vi "Experiment header-Save_Load config file data.vi"(5 "Header file actions":T1=enum."Write All", 7 "Header file sections":T19=enum."LOGIN", 8 "error in (no error)":errorcluster, 9 "All header parameters in":T2 {"VOLUME IMAGING"."Plane Mode" items=["XY Plane", "XZ Plane", "YZ Plane", "arbitraryplane"]; "VOLUME IMAGING"."Basic Image meta data"."Frame Size" items=["100X100"=100, "128X128"=128, "200X200"=200, "256X256"=256, "512X512"=512, "1024x1024"=1024, "2048x2048"=2048]; "AOL Z-STACK"."Hdr Basic Image meta data"."Frame Size" items=["100X100"=100, "128X128"=128, "200X200"=200, "256X256"=256, "512X512"=512, "1024x1024"=1024, "2048x2048"=2048]; "MOTOR Z-STACK"."Hdr Basic Image meta data"."Frame Size" items=["100X100"=100, "128X128"=128, "200X200"=200, "256X256"=256, "512X512"=512, "1024x1024"=1024, "2048x2048"=2048]; "FUNCTIONAL IMAGING"."Plane Mode" items=["XY Plane", "XZ Plane", "YZ Plane", "arbitraryplane"]; "FUNCTIONAL IMAGING"."Basic Image meta data"."Frame Size" items=["100X100"=100, "128X128"=128, "200X200"=200, "256X256"=256, "512X512"=512, "1024x1024"=1024, "2048x2048"=2048]; "TIME SERIES"."Basic Image meta data"."Frame Size" items=["100X100"=100, "128X128"=128, "200X200"=200, "256X256"=256, "512X512"=512, "1024x1024"=1024, "2048x2048"=2048]}, 11 "Experiment data folder path":path) -> (0 "error out":errorcluster, 1 "All header parameters out":T2 {"VOLUME IMAGING"."Plane Mode" items=["XY Plane", "XZ Plane", "YZ Plane", "arbitraryplane"]; "VOLUME IMAGING"."Basic Image meta data"."Frame Size" items=["100X100"=100, "128X128"=128, "200X200"=200, "256X256"=256, "512X512"=512, "1024x1024"=1024, "2048x2048"=2048]; "AOL Z-STACK"."Hdr Basic Image meta data"."Frame Size" items=["100X100"=100, "128X128"=128, "200X200"=200, "256X256"=256, "512X512"=512, "1024x1024"=1024, "2048x2048"=2048]; "MOTOR Z-STACK"."Hdr Basic Image meta data"."Frame Size" items=["100X100"=100, "128X128"=128, "200X200"=200, "256X256"=256, "512X512"=512, "1024x1024"=1024, "2048x2048"=2048]; "FUNCTIONAL IMAGING"."Plane Mode" items=["XY Plane", "XZ Plane", "YZ Plane", "arbitraryplane"]; "FUNCTIONAL IMAGING"."Basic Image meta data"."Frame Size" items=["100X100"=100, "128X128"=128, "200X200"=200, "256X256"=256, "512X512"=512, "1024x1024"=1024, "2048x2048"=2048]; "TIME SERIES"."Basic Image meta data"."Frame Size" items=["100X100"=100, "128X128"=128, "200X200"=200, "256X256"=256, "512X512"=512, "1024x1024"=1024, "2048x2048"=2048]})   [LabVIEW 2017]
doc: "This self-contained module handles all header files save/write operations.\nIt can generate a number of different header files containing different parameters.\nEach different type of header file has its own type defined cluster of parameters.\nThe functionality is fully self-scalable such as when new parameters are added or parameters are deleted or renamed in the typedef clusters this is all handled automatically without the need for further updates to this module."
uses:
  Typedefs/Header parameters cluster-ALL.ctl
  Typedefs/Header subclusters/Header params -Login.ctl
  Typedefs/Header subclusters/Header params-Global Parameters.ctl
  Misc/Experiment Type.ctl
  Typedefs/Header subclusters/Header params-Imaging Modes.ctl
  Typedefs/Header subclusters/Header params-Time Series.ctl
  Typedefs/Header subclusters/Header params-Basic image meta data.ctl
  Typedefs/Frame Size.ctl
  Typedefs/Header subclusters/Header params-Motor Z-stack.ctl
  Typedefs/Header subclusters/Header params-AOL Z-stack.ctl
  Typedefs/Header subclusters/Header params-Functional Imaging.ctl
  Typedefs/Functional Mode.ctl
  Typedefs/AOL modes.ctl
  Typedefs/Plane Mode.ctl
  Typedefs/Header subclusters/Header params-Calibration Setup.ctl
  Typedefs/Header subclusters/Header params-statistics.ctl
  Misc/Biology Information.ctl
  Typedefs/Header file sections.ctl
  Typedefs/Header file actions.ctl
panel:
  out "error":errorcluster
  # "Actual FOV ------>\n(not norm FOFV)"
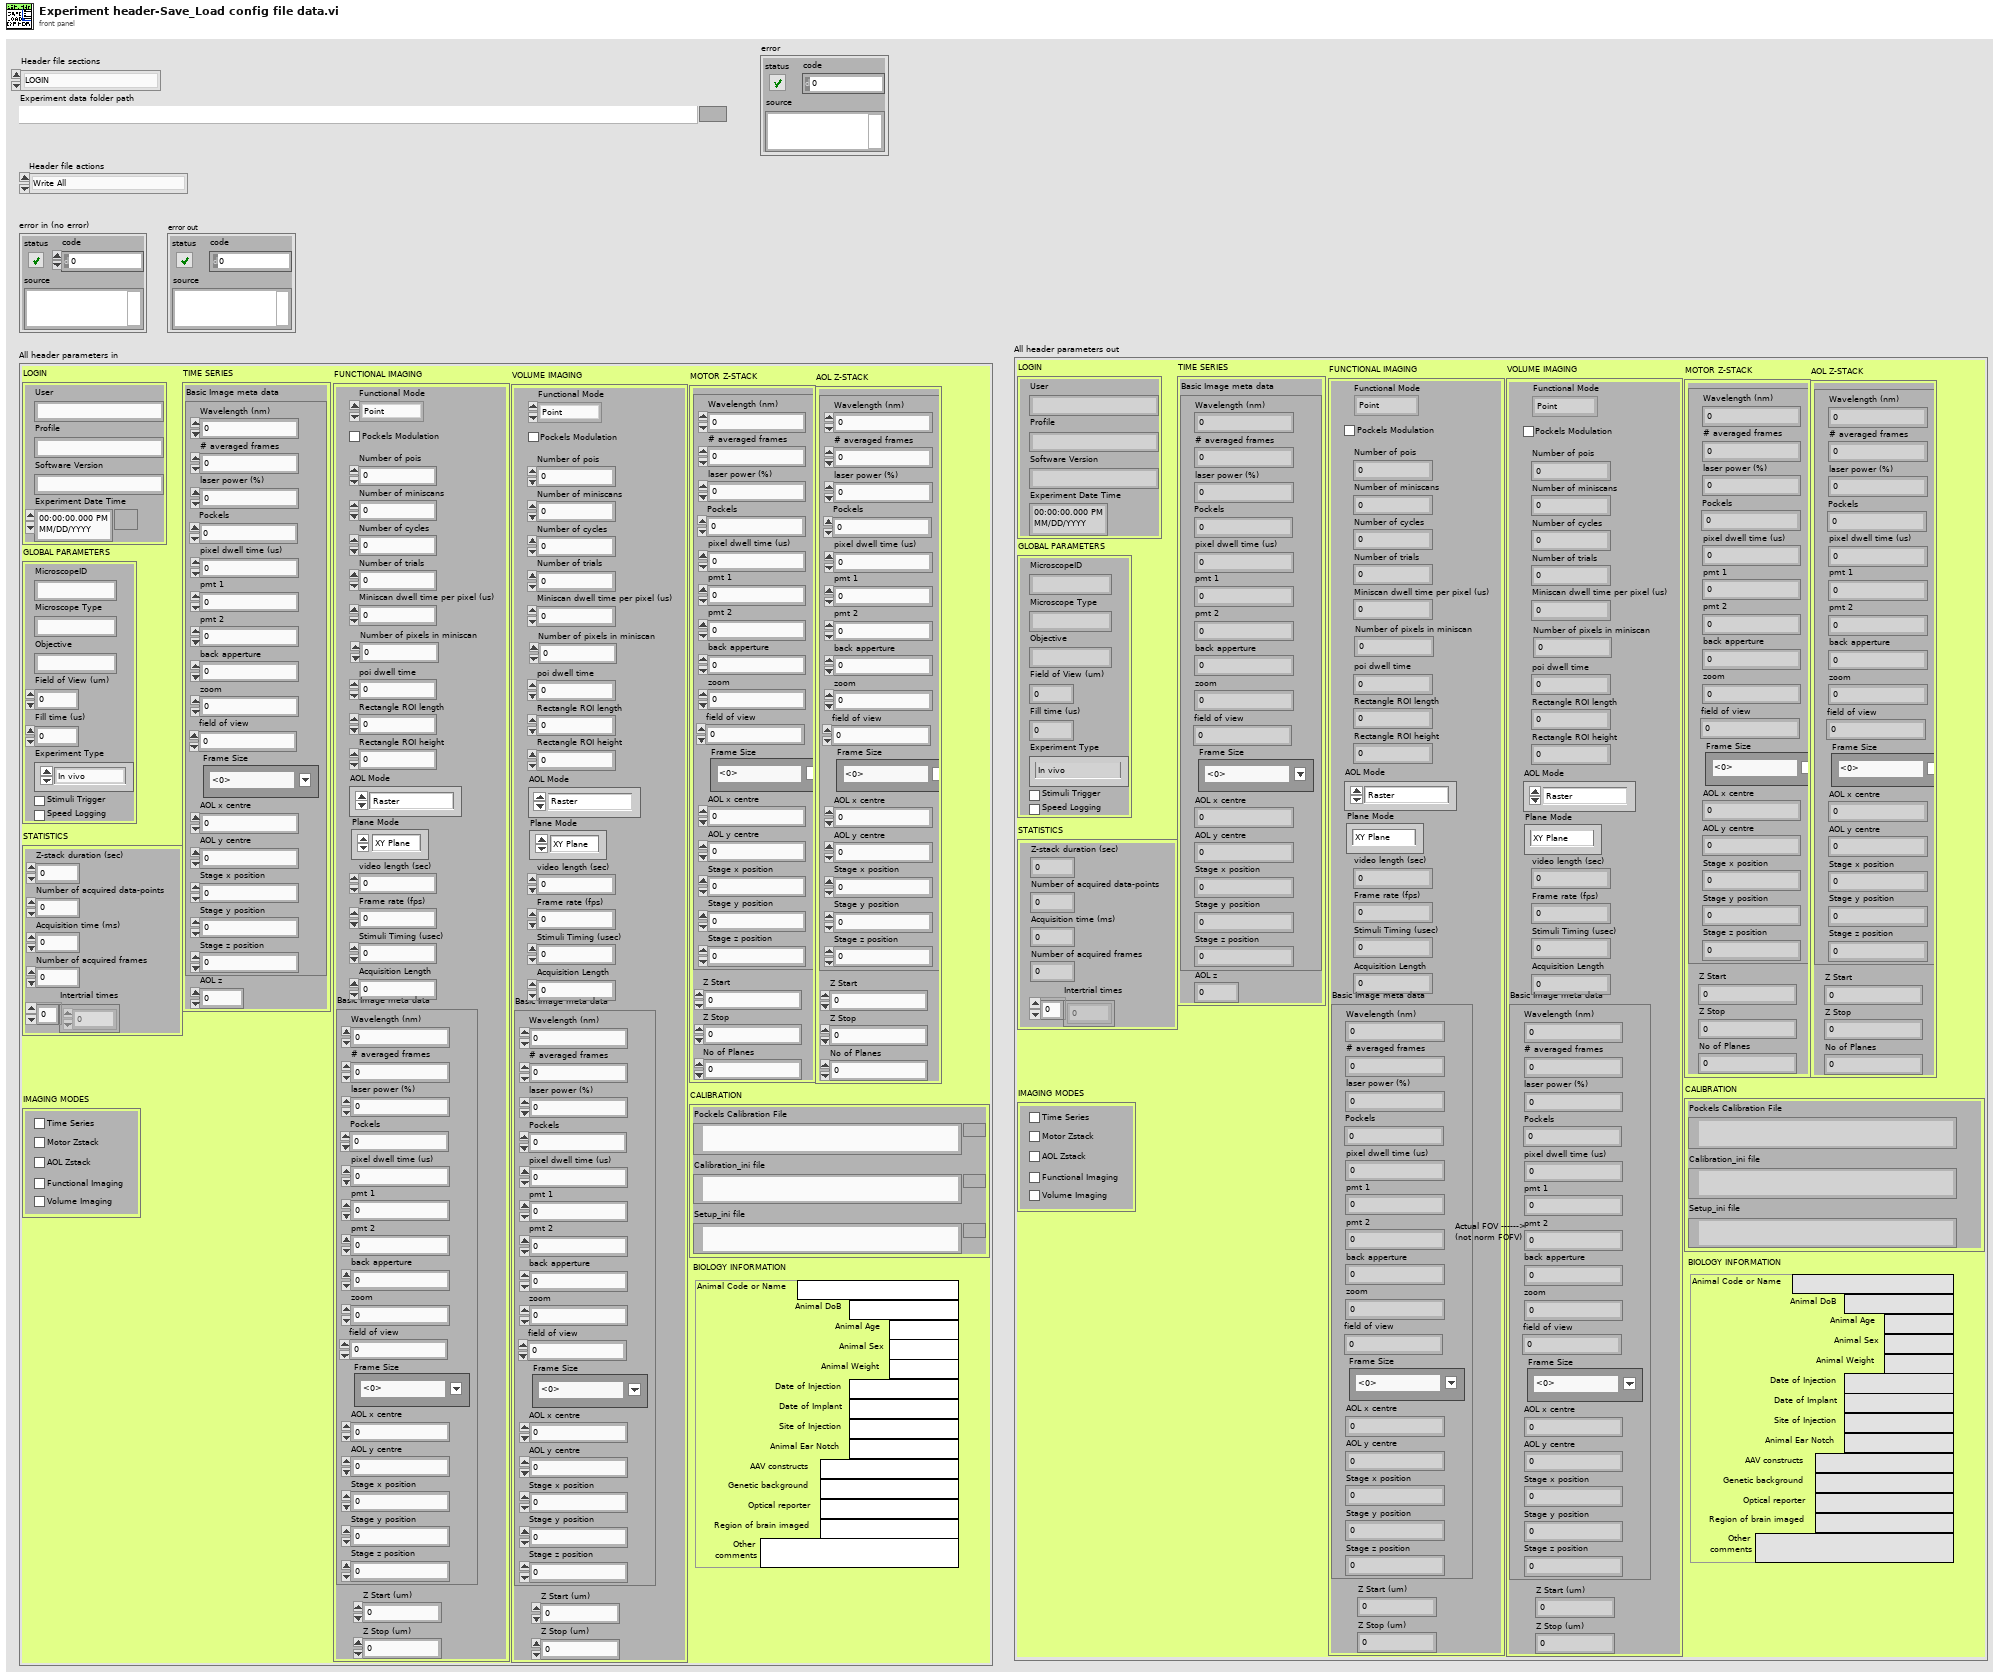
[diagram p1: front panel]
types:
  T1 = typedef "Header file actions.ctl" = enum16{"Create", "Open", "Read All", "Read Section", "Write All", "Write Section", "Close"}
  T2 = typedef "Header parameters cluster-ALL.ctl" = cluster{"LOGIN":T3, "GLOBAL PARAMETERS":T4, "IMAGING MODES":T6, "TIME SERIES":T7, "MOTOR Z-STACK ":T10, "AOL Z-STACK":T11, "FUNCTIONAL IMAGING":T12, "VOLUME IMAGING":T12, "CALIBRATION":T16, "STATISTICS":T17, "BIOLOGY INFORMATION":T18}
  T3 = typedef "Header params -Login.ctl" = cluster{"User":string, "Profile":string, "Software Version":string, "Experiment Date Time":timestamp}
  T4 = typedef "Header params-Global Parameters.ctl" = cluster{"MicroscopeID":string, "Microscope Type":string, "Objective":string, "Field of View (um)":dbl, "Fill time (us)":dbl, "Experiment Type":T5, "Stimuli Trigger":bool, "Speed Logging":bool}
  T5 = typedef "Experiment Type.ctl" = enum16{"In vivo", "In vitro", "Testing", "Calibration", "Other"}
  T6 = typedef "Header params-Imaging Modes.ctl" = cluster{"Time Series":bool, "Motor Zstack":bool, "AOL Zstack":bool, "Functional Imaging":bool, "Volume Imaging":bool}
  T7 = typedef "Header params-Time Series.ctl" = cluster{"Basic Image meta data":T8, "AOL z":dbl}
  T8 = typedef "Header params-Basic image meta data.ctl" = cluster{"Wavelength (nm)":dbl, "# averaged frames":dbl, "laser power (%)":dbl, "Pockels":dbl, "pixel dwell time (us)":dbl, "pmt 1":dbl, "pmt 2":dbl, "back apperture":dbl, "zoom":dbl, "field of view":dbl, "Frame Size":T9, "AOL x centre":dbl, "AOL y centre":dbl, "Stage x position":dbl, "Stage y position":dbl, "Stage z position":dbl}
  T9 = typedef "Frame Size.ctl" = u16
  T10 = typedef "Header params-Motor Z-stack.ctl" = cluster{"Hdr Basic Image meta data":T8, "Z Start":dbl, "Z Stop":dbl, "No of Planes":i32}
  T11 = typedef "Header params-AOL Z-stack.ctl" = cluster{"Hdr Basic Image meta data":T8, "Z Start":dbl, "Z Stop":dbl, "No of Planes":i32}
  T12 = typedef "Header params-Functional Imaging.ctl" = cluster{"Functional Mode":T13, "Pockels Modulation":bool, "Number of pois":dbl, "Number of miniscans":dbl, "Number of cycles":dbl, "Number of trials":dbl, "Miniscan dwell time per pixel (us)":dbl, "Number of pixels in miniscan":dbl, "poi dwell time":dbl, "Rectangle ROI length":dbl, "Rectangle ROI height":dbl, "AOL Mode":T14, "Plane Mode":T15, "video length (sec)":dbl, "Frame rate (fps)":dbl, "Stimuli Timing (usec)":dbl, "Acquisition Length":dbl, "Basic Image meta data":T8, "Z Start (um)":dbl, "Z Stop (um)":dbl}
  T13 = typedef "Functional Mode.ctl" = enum16{"Point", "Line", "Patch", "Plane", "Volume"}
  T14 = typedef "AOL modes.ctl" = enum16{"Raster", "Structural", "Pointing", "Mini Scan", "Alignment"}
  T15 = typedef "Plane Mode.ctl" = u16
  T16 = typedef "Header params-Calibration Setup.ctl" = cluster{"Pockels Calibration File":path, "Calibration_ini file":path, "Setup_ini file":path}
  T17 = typedef "Header params-statistics.ctl" = cluster{"Z-stack duration (sec)":dbl, "Number of acquired data-points":dbl, "Acquisition time (ms)":dbl, "Number of acquired frames":dbl, "Intertrial times":dbl[]}
  T18 = typedef "Biology Information.ctl" = cluster{"Animal Code or Name":string, "Animal DoB":string, "Animal Age":string, "Animal Sex":string, "Animal Weight":string, "Date of Injection":string, "Date of Implant":string, "Site of Injection":string, "Animal Ear Notch":string, "AAV constructs":string, "Genetic background":string, "Optical reporter":string, "Region of brain imaged":string, "Other \ncomments":string}
  T19 = typedef "Header file sections.ctl" = enum16{"ALL SECTIONS", "LOGIN", "GLOBAL PARAMETERS", "IMAGING MODES", "TIME SERIES", "MOTOR Z-STACK", "AOL Z-STACK", "FUNCTIONAL IMAGING", "VOLUME IMAGING", "CALIBRATION", "STATISTICS", "BIOLOGY INFORMATION"}
  T20 = typedef "Header file section refs.ctl" = cluster{"Section Name":string, "Section Ref":refnum<vi>, "Section Controls[]":refnum<vi>[]}
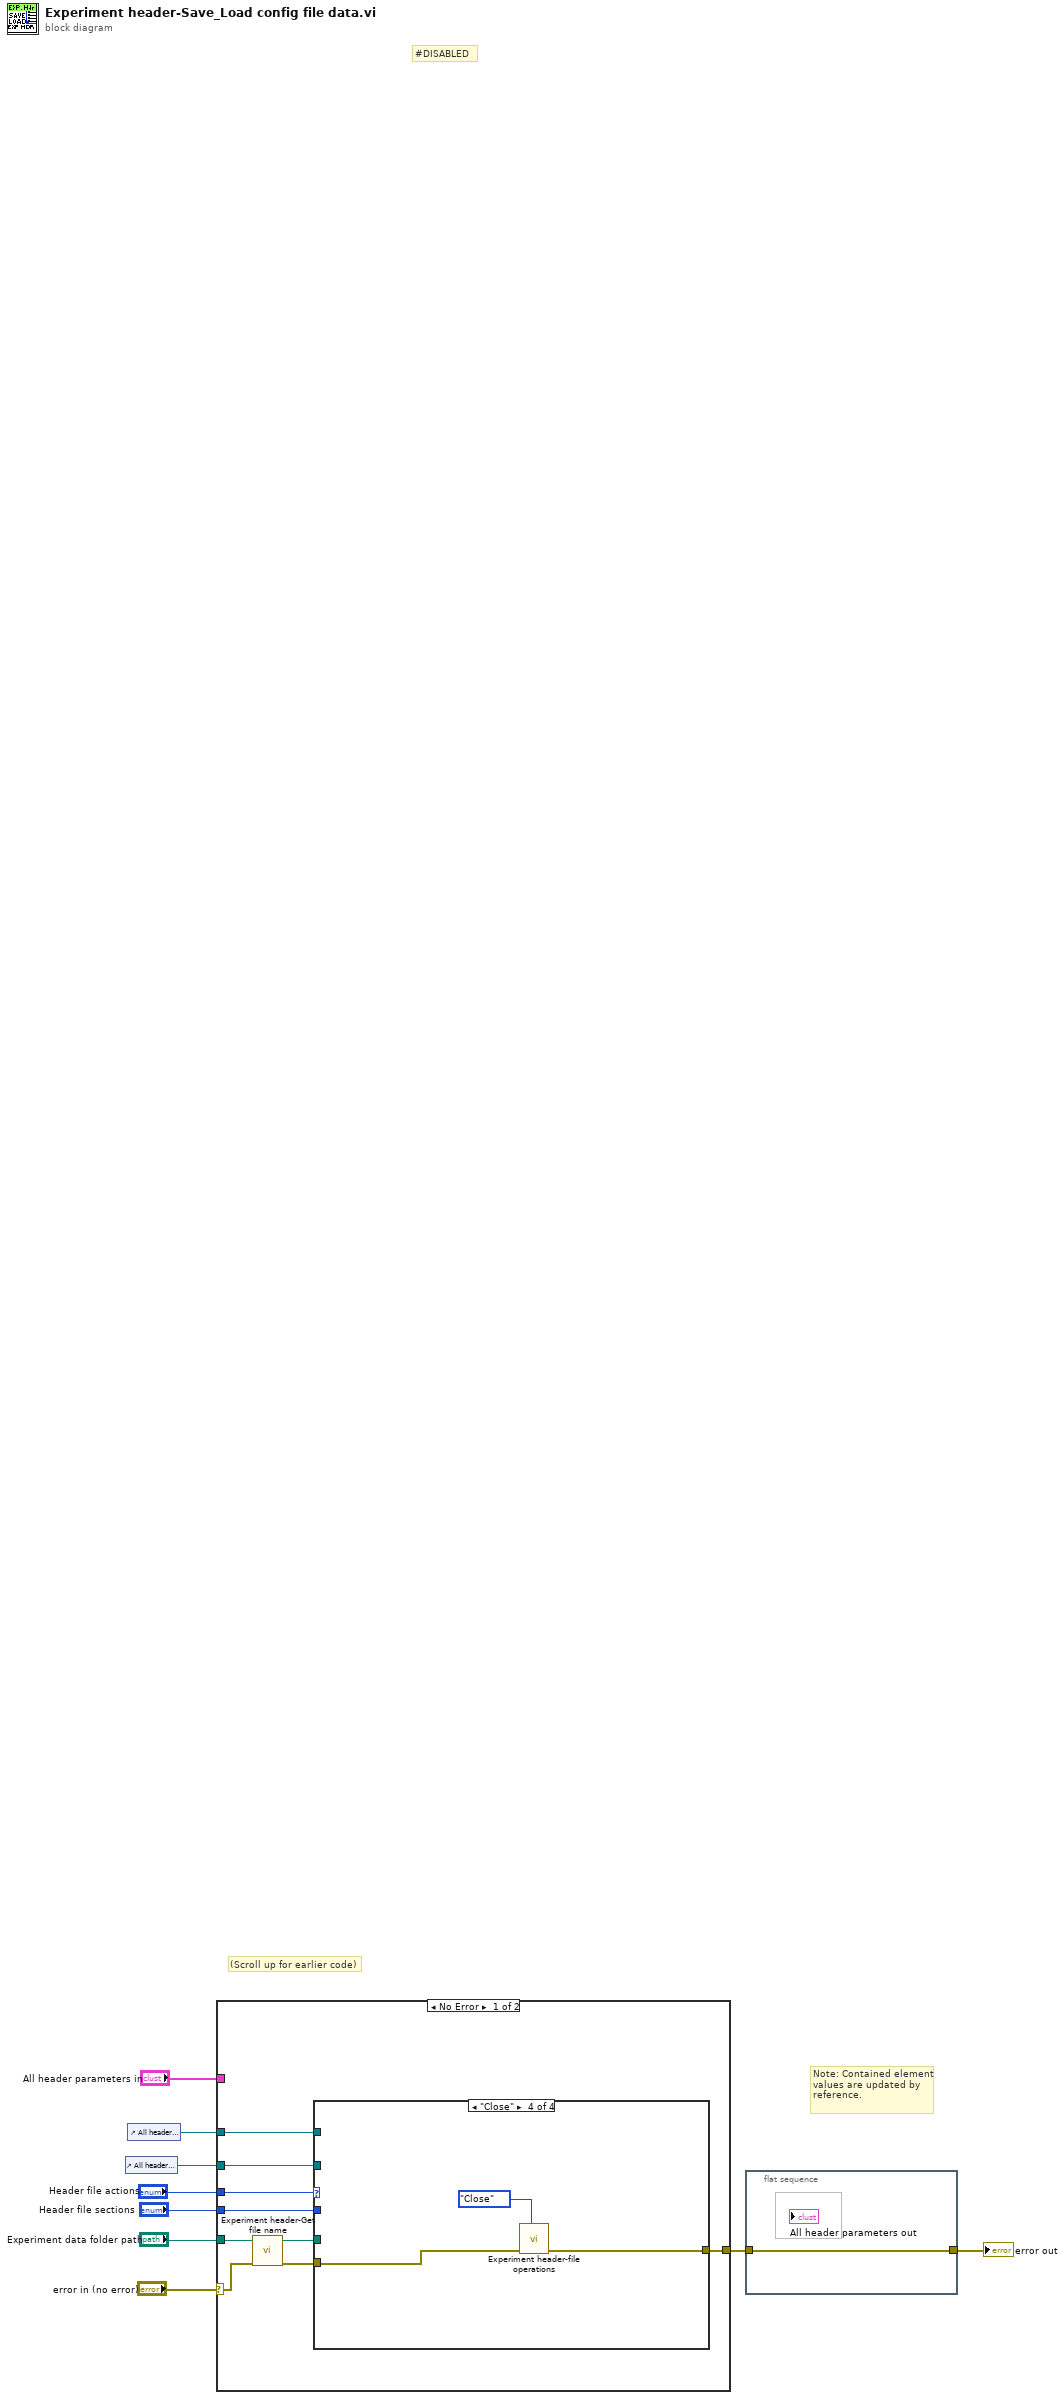
[diagram p0: block diagram]
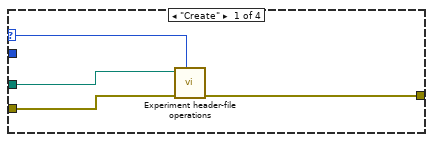
[diagram p2: hidden frame]
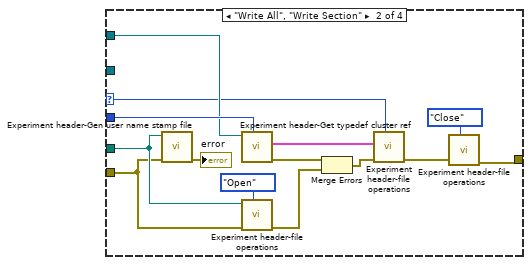
[diagram p3: hidden frame]
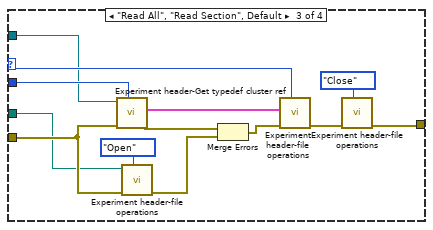
[diagram p4: hidden frame]
diagram:
  # "Note: Contained element values are updated by reference."
  # "(Scroll up for earlier code)"
  # "#DISABLED"
  n1 = control-ref of="All header parameters out"() -> (w3:refnum<vi>)
  n2 = control-ref of="All header parameters in"() -> (w4:refnum<vi>)
  n3 = case shown="No Error" "error in (no error)" {
    selector: "error in (no error)" -> [w11 w53]
    tunnel: [w10 w53] -> w2
    tunnel: "Header file sections" -> [w15 _]
    tunnel: "All header parameters in" -> [_ _]
    tunnel: "Experiment data folder path" -> [w18 _]
    tunnel: "Header file actions" -> [w14 _]
    tunnel: w4 -> [w13 _]
    tunnel: w3 -> [w12 _]
    frame No Error {
      n4 = call "Experiment header-Get file name.vi"("error in (no error)"=w11, "Experiment data folder path"=w18) -> ("error out"=w17:errorcluster, "Header File Path"=w16:path)  [unwired: 8 in]
      n5 = case shown="\"Close\"" w14 {
        selector: w14 -> [w21 w33 w48 _]
        tunnel: w17 -> [w22 w26 w44 w52]
        tunnel: w16 -> [w20 w32 w37 _]
        tunnel: w15 -> [_ w35 w47 _]
        tunnel: w13 -> [_ w34 _ _]
        tunnel: w12 -> [_ _ w46 _]
        tunnel: [w19 w23 w39 w50] -> w10
        frame "Create" {
          n6 = call "Experiment header-file operations.vi"("Header file actions"=w21, "error in (no error)"=w22, "Path"=w20) -> ("error out"=w19:errorcluster)  [unwired: 8 in]
        }
        frame "Write All", "Write Section" {
          n7 = call "Experiment header-Gen user name stamp file.vi"("error in (no error)"=w26, "Experiment data folder path"=w32) -> ("error out"=→"error":errorcluster)  [unwired: 9 in]
          n8 = call "Experiment header-Get typedef cluster ref.vi"("Header file sections"=w35, "All header parameters / Header module interface cluster"=w34) -> ("error out"=w30:errorcluster, "Section Refs"=w36:T20[])  [unwired: 6 in, 2 out]
          n9 = call "Experiment header-file operations.vi"("Header file actions"=Header_file_actions."Open", "error in (no error)"=w26, "Path"=w32) -> ("error out"=w29:errorcluster)  [unwired: 8 in]
          n10 = Merge Errors(w30, w29) -> (w28:errorcluster)
          n11 = call "Experiment header-file operations.vi"("Header file actions"=w33, "error in (no error)"=w28, "Section Refs"=w36) -> ("error out"=w24:errorcluster)  [unwired: 8 in]
          n12 = call "Experiment header-file operations.vi"("Header file actions"=Header_file_actions."Close", "error in (no error)"=w24) -> ("error out"=w23:errorcluster)  [unwired: 9 in]
        }
        frame "Read All", "Read Section", Default {
          n13 = call "Experiment header-Get typedef cluster ref.vi"("Header file sections"=w47, "error in (no error)"=w44, "All header parameters / Header module interface cluster"=w46) -> ("error out"=w43:errorcluster, "Section Refs"=w49:T20[])  [unwired: 5 in, 2 out]
          n14 = call "Experiment header-file operations.vi"("Header file actions"=Header_file_actions."Open", "error in (no error)"=w44, "Path"=w37) -> ("error out"=w41:errorcluster)  [unwired: 8 in]
          n15 = Merge Errors(w43, w41) -> (w42:errorcluster)
          n16 = call "Experiment header-file operations.vi"("Header file actions"=w48, "error in (no error)"=w42, "Section Refs"=w49) -> ("error out"=w38:errorcluster)  [unwired: 8 in]
          n17 = call "Experiment header-file operations.vi"("Header file actions"=Header_file_actions."Close", "error in (no error)"=w38) -> ("error out"=w39:errorcluster)  [unwired: 9 in]
        }
        frame "Close" {
          n18 = call "Experiment header-file operations.vi"("Header file actions"=Header_file_actions."Close", "error in (no error)"=w52) -> ("error out"=w50:errorcluster)  [unwired: 9 in]
        }
      }
    }
    frame Error {
    }
  }
  n19 = flat-sequence {
    tunnel: w2 -> [w54]
    tunnel: [w54] -> w1
    frame #0 {
    }
  }
  "error out" <- w1
